vi "Get Temperature.vi"(7 "VISA resource":refnum<visa-resource-name>, 8 "error in (no error)":errorcluster, 9 "Name":string, 10 "Data":T1={"Record heater"=FALSE, "Record RAW"=FALSE, "Set point"=0.0, "Heater range"=0.0, "Approach"=enum."Instant", "Ramp rate, K/min"=1.0, "Record Channels"=[], "Settling time "=60.0, "Settling range"=0.1, "P"=0.0, "I"=0.0, "D"=0.0, "Temperature Control"=FALSE}, 11 "Neocera in":refnum<class "Neocera.lvclass">) -> (0 "error out":errorcluster, 1 "Channel data":dbl[](array[numeric]), 2 "Channel names":string[](array[string]), 3 "Neocera out":refnum<class "Neocera.lvclass">, 4 "Controled temperature":dbl, 5 "VISA resource out":refnum<visa-resource-name>)   [LabVIEW 2015, in "Neocera.lvclass"]
uses:
  Neocera.lvclass
  Temperarture Controller/T controller parameters.ctl
  Instruments/Neocera/Neocera Set Point Aproach.ctl
panel:
  out "Heat %":dbl format="%.2f"
  # "Temperature Monitor"
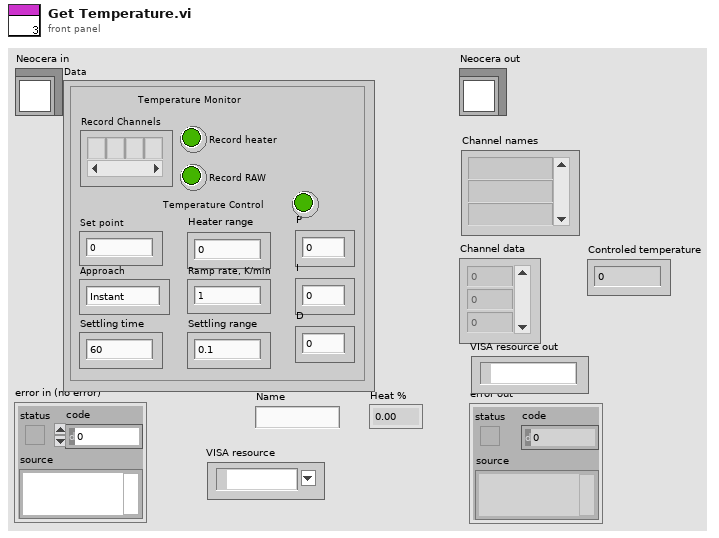
[diagram p1: front panel]
types:
  T1 = typedef "T controller parameters.ctl" = cluster{"Record heater":bool, "Record RAW":bool, "Set point":dbl, "Heater range":dbl, "Approach":T2, "Ramp rate, K/min":dbl, "Record Channels":string[], "Settling time ":dbl, "Settling range":dbl, "P":dbl, "I":dbl, "D":dbl, "Temperature Control":bool}
  T2 = typedef "Neocera Set Point Aproach.ctl" = enum16{"Instant", "Ramp"}
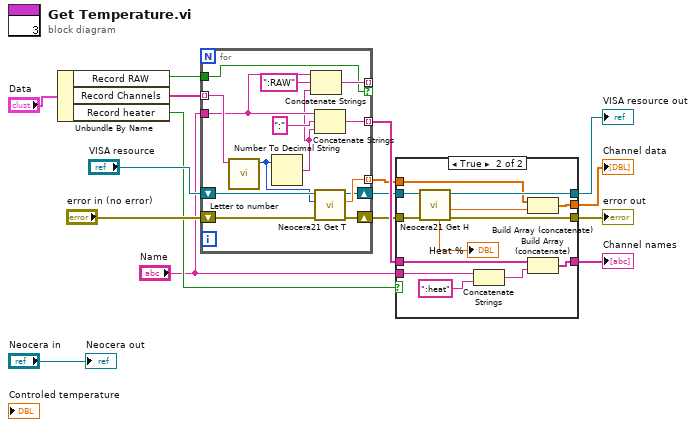
[diagram p0: block diagram]
diagram:
  n1 = Unbundle By Name("Data") -> ("Record RAW"=w1:bool, "Record Channels"=w13:string[], "Record heater"=w11:bool)
  n2 = for {
    tunnel: [w26] -> w5 mode=indexing
    shift-right: [w25] -> w9
    shift-left: "VISA resource" -> [w29]
    shift-right: [w27] -> w8
    shift-left: "error in (no error)" -> [w28]
    tunnel: w13 -> [w24] mode=indexing
    tunnel: "Name" -> [w21]
    tunnel: [w30] -> w10 mode=indexing
    tunnel: [w18] -> _ mode=indexing if=w17
    tunnel: w1 -> [w17]
    n3 = call "Letter to number.vi"("String"=w24) -> ("Number"=w23:i32)  [unwired: 10 in]
    n4 = Number To Decimal String(number=w23) -> (decimal integer string=w19:string)  [unwired: 1 in]
    n5 = Concatenate Strings(w21, ":RAW" ("string"), w19) -> (w18:string)
    n6 = Concatenate Strings(w21, ":" ("string"), w19) -> (w30:string)
    n7 = call "Neocera21 Get T.vi"("error in (no error)"=w28, "Sensor"=w23, "VISA Resource Name"=w29) -> ("error out"=w27:errorcluster, "Temperature"=w26:dbl, "VISA Resource Name Out"=w25:refnum<visa-resource-name>)  [unwired: 5 in, 1 out]
  }
  n8 = case shown="True" w11 {
    tunnel: w8 -> [w34 w40]
    tunnel: [w34 w47] -> w7
    tunnel: w9 -> [w33 w41]
    tunnel: [w33 w46] -> w2
    tunnel: w10 -> [w32 w45]
    tunnel: [w32 w44] -> w3
    tunnel: w5 -> [w31 w43]
    tunnel: [w31 w42] -> w6
    tunnel: "Name" -> [_ w37]
    frame False {
    }
    frame True {
      n9 = call "Neocera21 Get H.vi"("error in (no error)"=w40, "VISA Resource Name"=w41) -> ("error out"=w47:errorcluster, "Heater power"=w39:dbl, "VISA Resource Name Out"=w46:refnum<visa-resource-name>, "Heat %"=→"Heat %":dbl)  [unwired: 4 in, 2 out]
      n10 = Concatenate Strings(w37, ":heat" ("string")) -> (w35:string)
      n11 = Build Array (concatenate)(w43, w39) -> (w42:dbl[])
      n12 = Build Array (concatenate)(w45, w35) -> (w44:string[])
    }
  }
  "error out" <- w7
  "VISA resource out" <- w2
  "Channel data" <- w6
  "Channel names" <- w3
  "Neocera out" <- "Neocera in"
